vi "_API_BINANCE_POST_USDT_FEATURES_changeInitialLeverage.vi"(0 "BinanceAPI in":refnum<class "BinanceAPI_.lvclass">, 5 "Change Initial Leverage":T1={"symbol (eg. BTCUSDT)"="CAKEUSDT", "leverage"=1, "recvWindow"=5000}, 11 "error in (no error)":errorcluster) -> (4 "BinanceAPI out":refnum<class "BinanceAPI_.lvclass">, 14 "Body":string, 15 "error out":errorcluster)   [LabVIEW 2022 SP3, in "BinanceAPI_.lvclass"]
doc: "https://binance-docs.github.io/apidocs/futures/en/#change-initial-leverage-trade"
uses:
  BinanceAPI_.lvclass
  BinanceAPI_.lvclass/BinanceAPI_.ctl
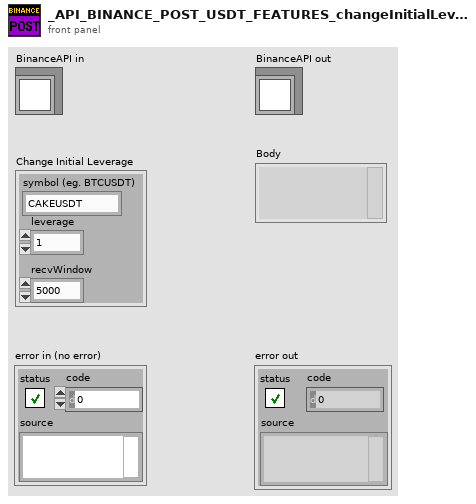
[diagram p1: front panel]
types:
  T1 = cluster{"symbol (eg. BTCUSDT)":string, "leverage":i8, "recvWindow":i32}
  T2 = enum16{"SPOT", "USDT_FUTURES", "COIN_FUTURES", "VANILLA"}
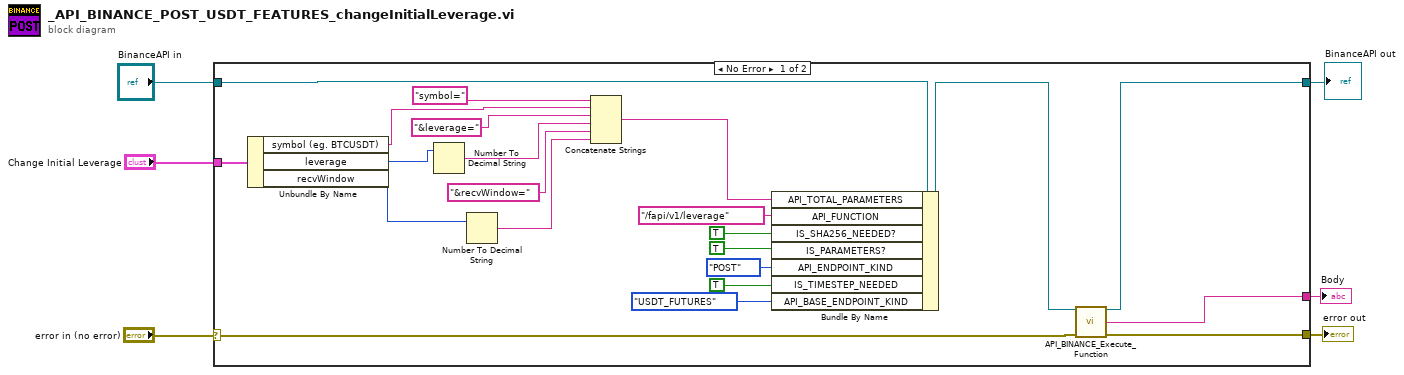
[diagram p0: block diagram]
diagram:
  n1 = case shown="No Error" "error in (no error)" {
    selector: "error in (no error)" -> [w19 w30]
    tunnel: [w15 w30] -> w5
    tunnel: [w16 w29] -> w1
    tunnel: "BinanceAPI in" -> [w20 w29]
    tunnel: "Change Initial Leverage" -> [w25 _]
    tunnel: [w7 _] -> w3
    frame No Error {
      n2 = Unbundle By Name(w25) -> ("symbol (eg. BTCUSDT)"=w22:string, "leverage"=w11:i8, "recvWindow"=w13:i32)
      n3 = Number To Decimal String(number=w11) -> (decimal integer string=w10:string)  [unwired: 1 in]
      n4 = Number To Decimal String(number=w13) -> (decimal integer string=w8:string)  [unwired: 1 in]
      n5 = Concatenate Strings("symbol=" ("Symbol"), w22, "&leverage=" ("Symbol"), w10, "&recvWindow=" ("Symbol"), w8) -> (w24:string)
      n6 = Bundle By Name(cluster=w20, "API_TOTAL_PARAMETERS"=w24, "API_FUNCTION"="/fapi/v1/leverage", "IS_SHA256_NEEDED?"=TRUE, "IS_PARAMETERS?"=TRUE, "API_ENDPOINT_KIND"=enum16{"POST", "DELETE", "GET", "PUT"}."POST", "IS_TIMESTEP_NEEDED"=TRUE ("IS_PARAMETERS?"), "API_BASE_ENDPOINT_KIND"=T2."USDT_FUTURES") -> (w17:refnum<class "BinanceAPI_.lvclass">)
      n7 = call "API_BINANCE_Execute_Function.vi"("BinanceAPI in"=w17, "error in (no error)"=w19) -> ("BinanceAPI out"=w16:refnum<class "BinanceAPI_.lvclass">, "Body"=w7:string, "error out"=w15:errorcluster)  [unwired: 9 in, 2 out]
    }
    frame Error {
    }
  }
  "error out" <- w5
  "Body" <- w3
  "BinanceAPI out" <- w1
